vi "WaveformGraph.vi"(8 "error in":errorcluster, 11 "Gen Refnum":refnum<vi>) -> (0 "error out":errorcluster, 3 "WFGraph out":refnum<class "WaveformGraph.lvclass">)   [LabVIEW 2014, in "WaveformGraph.lvclass"]
uses:
  WaveformGraph.lvclass
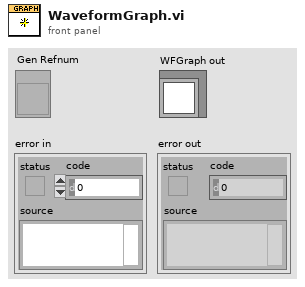
[diagram p1: front panel]
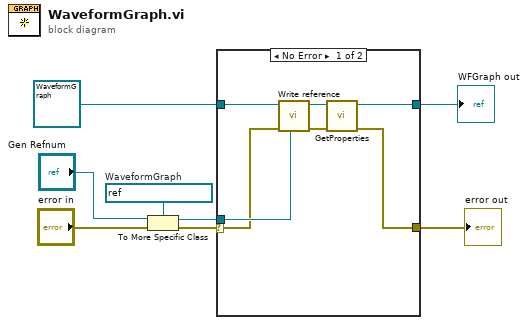
[diagram p0: block diagram]
diagram:
  w5 = refnum<vi> refnum  # WaveformGraph
  n1 = To More Specific Class(target class=w5, reference="Gen Refnum", error in="error in") -> (specific class reference=w2:refnum<vi>, error out=w3:errorcluster)
  n2 = case shown="No Error" w3 {
    selector: w3 -> [w13 w17]
    tunnel: w2 -> [w14 _]
    tunnel: refnum<class "WaveformGraph.lvclass"> refnum ("Scale in") -> [w15 w16]
    tunnel: [w9 w17] -> w6
    tunnel: [w11 w16] -> w7
    frame No Error {
      n3 = call-dynamic "Write reference.vi"("reference"=w14, "error in"=w13, "GObject in"=w15) -> ("error out"=w10:errorcluster, "GObject out"=w12:refnum<class "WaveformGraph.lvclass">)  [unwired: 5 in]
      n4 = call-dynamic "GetProperties.vi"("error in"=w10, "WaveformChart in"=w12) -> ("error out"=w9:errorcluster, "WaveformChart out"=w11:refnum<class "WaveformGraph.lvclass">)  [unwired: 8 in]
    }
    frame Error {
    }
  }
  "error out" <- w6
  "WFGraph out" <- w7
